vi "Analysis Configuration Dialog.vi"(11 "Data in":T1={"UI References"={"Exit Ref"=refnum, "Save Ref"=refnum, "Open Ref"=refnum, "Export Ref"=refnum, "Acquire Ref"=refnum, "Configure Ref"=refnum, "Graph Ref"=refnum, "Clear Ref"=refnum, "Analyze Ref"=refnum, "Status Ref"=refnum, "Snapshot Ref"=refnum}, "Graph Data"={"Data"=[], "Annotation List"=[], "Cursor List"=[], "Analysis Data"=[]}, "User Specified"={"Hardware Configuration"={"HW Refnum <Replace Me>"="", "Signal Type <Replace Me>"=enum."Sine Wave"}, "Analysis Configuration"={"Statistics"=TRUE}, "New Data Behavior"=enum."Replace"}}) -> (3 "Data out":T1={"UI References"={"Exit Ref"=refnum, "Save Ref"=refnum, "Open Ref"=refnum, "Export Ref"=refnum, "Acquire Ref"=refnum, "Configure Ref"=refnum, "Graph Ref"=refnum, "Clear Ref"=refnum, "Analyze Ref"=refnum, "Status Ref"=refnum, "Snapshot Ref"=refnum}, "Graph Data"={"Data"=[], "Annotation List"=[], "Cursor List"=[], "Analysis Data"=[]}, "User Specified"={"Hardware Configuration"={"HW Refnum <Replace Me>"="", "Signal Type <Replace Me>"=enum."Sine Wave"}, "Analysis Configuration"={"Statistics"=TRUE}, "New Data Behavior"=enum."Replace"}})   [LabVIEW 2023]
doc: "Displays the analysis configuration dialog if the user has the \"Prompt?\" preference set."
uses:
  controls/Data.ctl
  controls/UI References.ctl
  controls/Graph Data.ctl
  <vilib>/Utility/miscctls.llb/LVAnnotationListTypeDef.ctl
  <vilib>/Utility/miscctls.llb/LVCursorListTypeDef.ctl
  controls/User Specified Data.ctl
  controls/HW Configuration.ctl
  controls/Simulated Signal Type.ctl
  controls/Analysis Configuration.ctl
  controls/New Data Behavior.ctl
panel:
  # "(Scroll up to see large state data in/out clusters)"
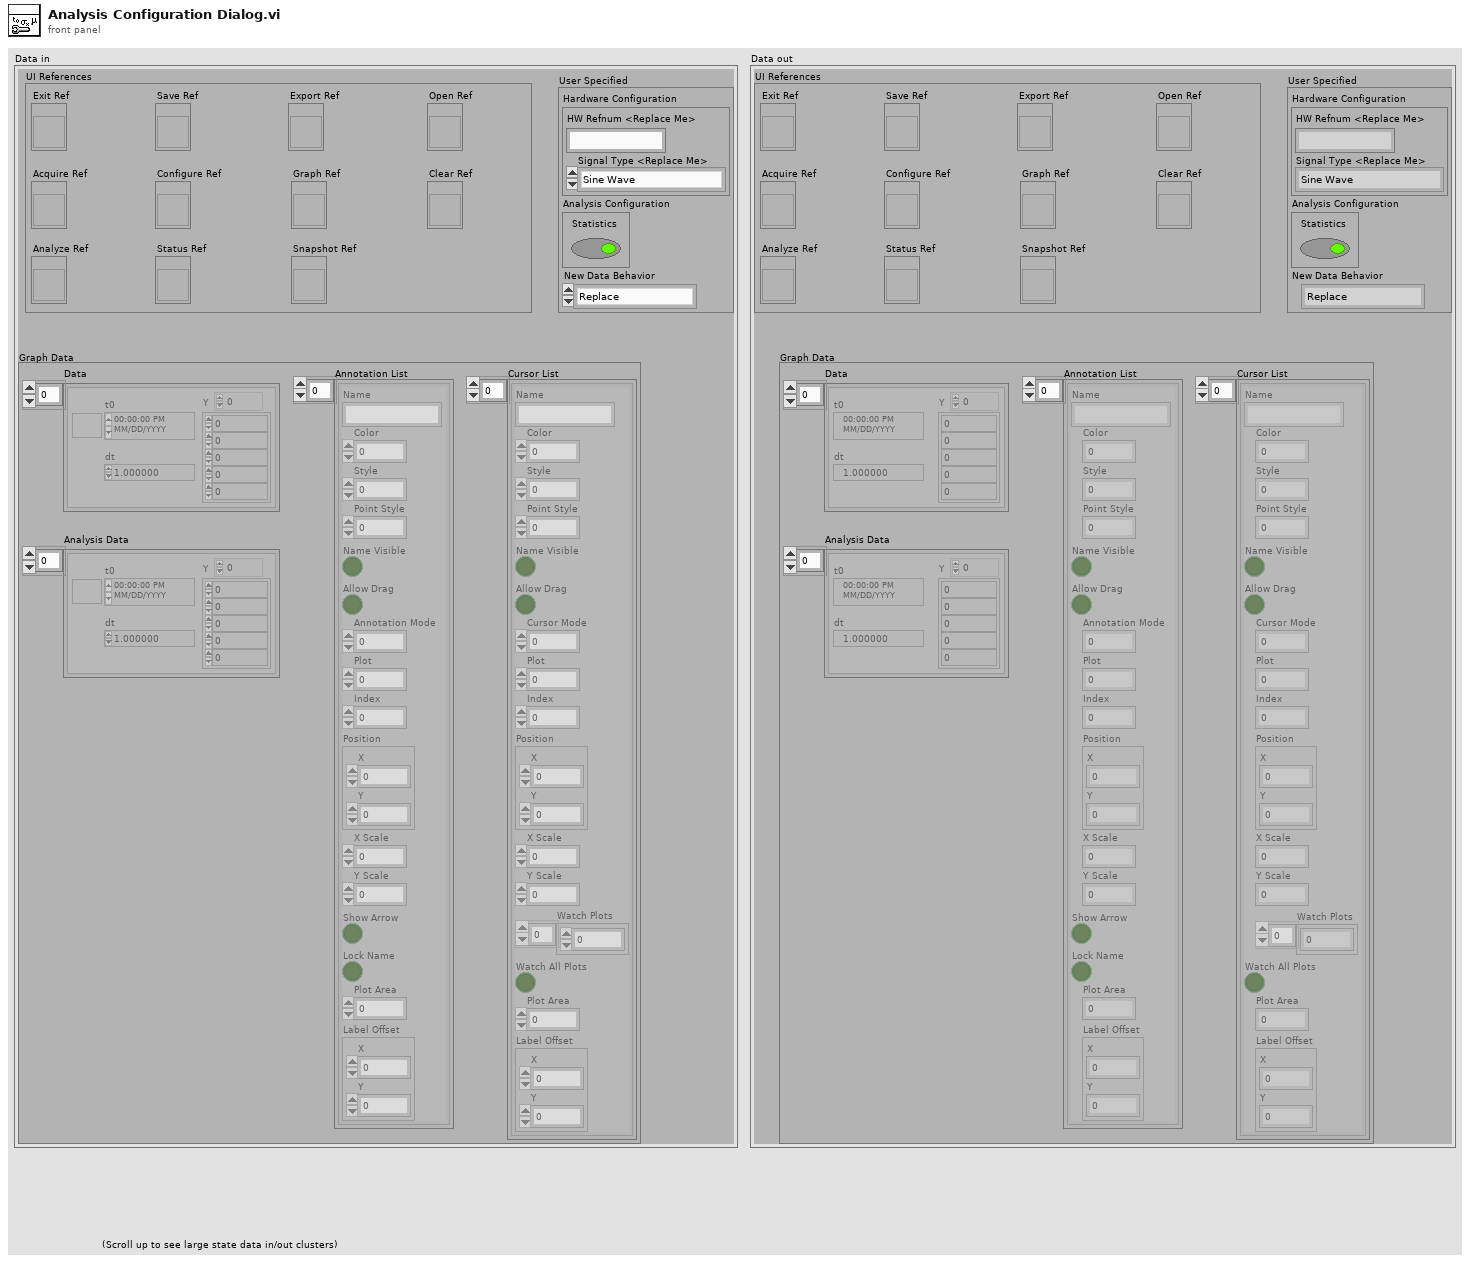
[diagram p1: front panel]
types:
  T1 = typedef "Data.ctl" = cluster{"UI References":T2, "Graph Data":T3, "User Specified":T6}
  T2 = typedef "UI References.ctl" = cluster{"Exit Ref":refnum<vi>, "Save Ref":refnum<vi>, "Open Ref":refnum<vi>, "Export Ref":refnum<vi>, "Acquire Ref":refnum<vi>, "Configure Ref":refnum<vi>, "Graph Ref":refnum<vi>, "Clear Ref":refnum<vi>, "Analyze Ref":refnum<vi>, "Status Ref":refnum<vi>, "Snapshot Ref":refnum<vi>}
  T3 = typedef "Graph Data.ctl" = cluster{"Data":waveform(dbl)[], "Annotation List":T4, "Cursor List":T5, "Analysis Data":waveform(dbl)[]}
  T4 = typedef "LVAnnotationListTypeDef.ctl" = cluster{"Name":string, "Color":u32, "Style":u8, "Point Style":u8, "Name Visible":bool, "Allow Drag":bool, "Annotation Mode":u32, "Plot":i32, "Index":i32, "Position":cluster{"X":dbl, "Y":dbl}, "X Scale":u32, "Y Scale":u32, "Show Arrow":bool, "Lock Name":bool, "Plot Area":i32, "Label Offset":cluster{"X":dbl, "Y":dbl}}[]
  T5 = typedef "LVCursorListTypeDef.ctl" = cluster{"Name":string, "Color":u32, "Style":u8, "Point Style":u8, "Name Visible":bool, "Allow Drag":bool, "Cursor Mode":u32, "Plot":i32, "Index":i32, "Position":cluster{"X":dbl, "Y":dbl}, "X Scale":u32, "Y Scale":u32, "Watch Plots":i32[], "Watch All Plots":bool, "Plot Area":i32, "Label Offset":cluster{"X":dbl, "Y":dbl}}[]
  T6 = typedef "User Specified Data.ctl" = cluster{"Hardware Configuration":T7, "Analysis Configuration":T9, "New Data Behavior":T10}
  T7 = typedef "HW Configuration.ctl" = cluster{"HW Refnum <Replace Me>":string, "Signal Type <Replace Me>":T8}
  T8 = typedef "Simulated Signal Type.ctl" = enum16{"Sine Wave", "Square Wave"}
  T9 = typedef "Analysis Configuration.ctl" = cluster{"Statistics":bool}
  T10 = typedef "New Data Behavior.ctl" = enum16{"Replace", "Overlay", "Append"}
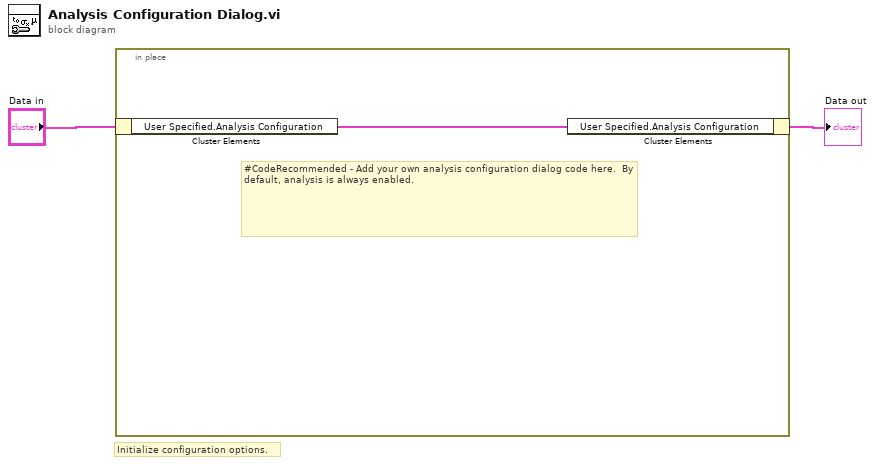
[diagram p0: block diagram]
diagram:
  # "Initialize configuration options."
  n1 = in-place {
    # "#CodeRecommended - Add your own analysis configuration dialog code here.  By default, analysis is always enabled."
    n2 = in-place-cluster #1("Data in") -> ("User Specified.Analysis Configuration"=w3:T9)
    n3 = in-place-cluster #1("User Specified.Analysis Configuration"=w3) -> (→"Data out":T1)
  }
